vi "启动.vi"() -> ()   [LabVIEW 2015, in "多对一启动器.lvlib"]
uses:
  <vilib>/ActorFramework/Actor/Actor.lvclass
  <vilib>/Instr/_visa.llb/VISA Configure Serial Port (Instr).vi
panel:
  in  "客户端COM":refnum<visa-resource-name>="COM29"
  in  "硬件COM":refnum<visa-resource-name>="COM30"
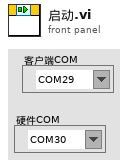
[diagram p1: front panel]
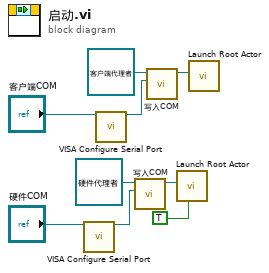
[diagram p0: block diagram]
diagram:
  n1 = call-poly "VISA Configure Serial Port"("VISA resource name"="硬件COM") -> ("VISA resource name out"=w2:refnum<visa-resource-name>)  [unwired: 13 in, 1 out]
  n2 = call-poly "VISA Configure Serial Port"("VISA resource name"="客户端COM") -> ("VISA resource name out"=w4:refnum<visa-resource-name>)  [unwired: 13 in, 1 out]
  n3 = call-dynamic "写入COM.vi"("COM"=w2, "通讯输入"=refnum<class "硬件代理者.lvclass"> refnum ("硬件代理者.lvlib:硬件代理者.lvclass")) -> ("通讯输出"=w6:refnum<class "硬件代理者.lvclass">)  [unwired: 8 in, 1 out]
  n4 = call-dynamic "写入COM.vi"("COM"=w4, "通讯输入"=refnum<class "客户端代理者.lvclass"> refnum ("客户端代理者.lvlib:客户端代理者.lvclass")) -> ("通讯输出"=w7:refnum<class "客户端代理者.lvclass">)  [unwired: 8 in, 1 out]
  n5 = call <vilib>:"Launch Root Actor.vi"("Open Actor Core front panel? (F)"=TRUE, "Actor"=w6) -> ()  [unwired: 8 in, 2 out]
  n6 = call <vilib>:"Launch Root Actor.vi"("Actor"=w7) -> ()  [unwired: 9 in, 2 out]
